vi "UTIL - ElapsedTime.vi"(8 "error in":errorcluster) -> (0 "error out":errorcluster, 2 "Elapsed (ms)":u32, 3 "ms value":u32)   [LabVIEW 2015, in "niDTS CommLib.lvlib" / "niDTS Comm String.lvclass"]
uses:
  niDTS Comm String.lvclass
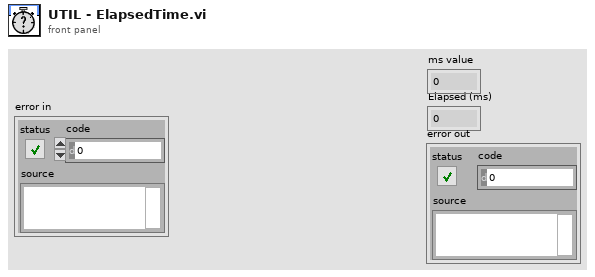
[diagram p1: front panel]
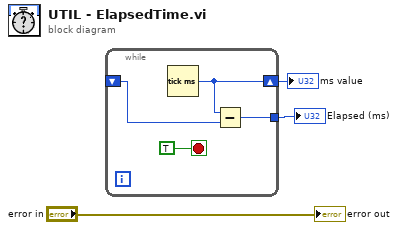
[diagram p0: block diagram]
diagram:
  n1 = while {
    shift-right: [w6] -> w1
    shift-left: _ -> [w5]
    tunnel: [w4] -> w3
    stop <- TRUE stop-if-true
    n2 = Tick Count (ms)() -> (millisecond timer value=w6:u32)
    n3 = Subtract(x=w6, y=w5) -> (x-y=w4:u32)
  }
  "Elapsed (ms)" <- w3
  "ms value" <- w1
  "error out" <- "error in"
